vi "addTagToTree.vi"(0 "Tree ref":refnum<vi>, 1 "Element name":string, 2 "Calibration path":string, 3 "Stimulus path":string, 5 "parent tag":string, 7 "Child Position":i32=-1, 9 "new tag":string, 11 "Symbol":i32=20, 12 "Req":string, 13 "Req doc path":string, 14 "Analysis script path":string) -> (6 "New Element Tag":string)   [LabVIEW 2010]
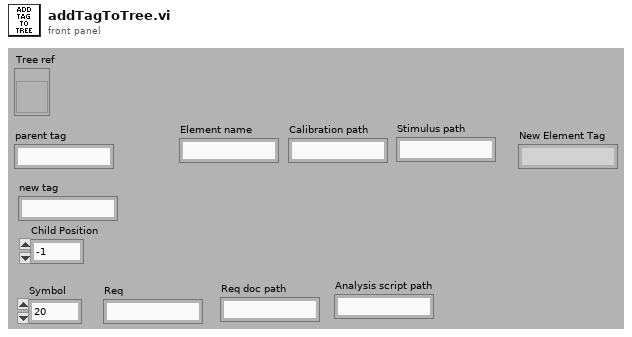
[diagram p1: front panel]
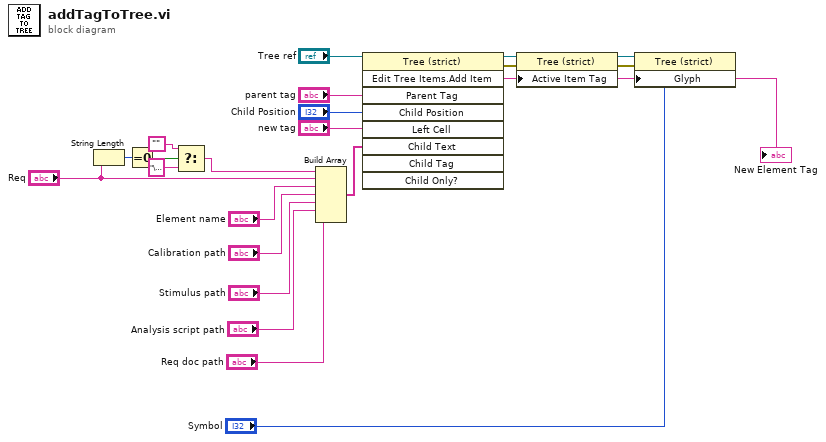
[diagram p0: block diagram]
diagram:
  n1 = String Length(string="Req") -> (length=w5:i32)
  n2 = Equal To 0?(x=w5) -> (x = 0?=w4:bool)
  n3 = Select(t="", s=w4, f="\u0007") -> (s? t:f=w1:string)
  n4 = Build Array(w1, "Req", "Element name", "Calibration path", "Stimulus path", "Analysis script path", "Req doc path") -> (w12:string[])
  n5 = invoke on="Invoke Node" class="Tree (strict)" method="Edit Tree Items.Add Item"(reference="Tree ref", "Parent Tag"="parent tag", "Child Position"="Child Position", "Left Cell"="new tag", "Child Text"=w12) -> (reference out=w19:refnum<vi>, error out=w17:errorcluster, "Edit Tree Items:Add Item"=w16:string)  [unwired: 4 in, 6 out]
  "New Element Tag" <- w16
  n6 = property on="Property Node" class="Tree (strict)"(reference=w19, error in=w17, "Active Item Tag"=w16) -> (reference out=w20:refnum<vi>, error out=w14:errorcluster)
  n7 = property on="Property Node" class="Tree (strict)"(reference=w20, error in=w14, "Glyph"="Symbol") -> ()  [unwired: 2 out]
